vi "Roi_test.vi"() -> ()   [LabVIEW 2021]
panel:
  in  "Combo Box":string(combo)
  out "Image 2":T1(plugin-control)
  in  "stop":bool
  in  "input image":path
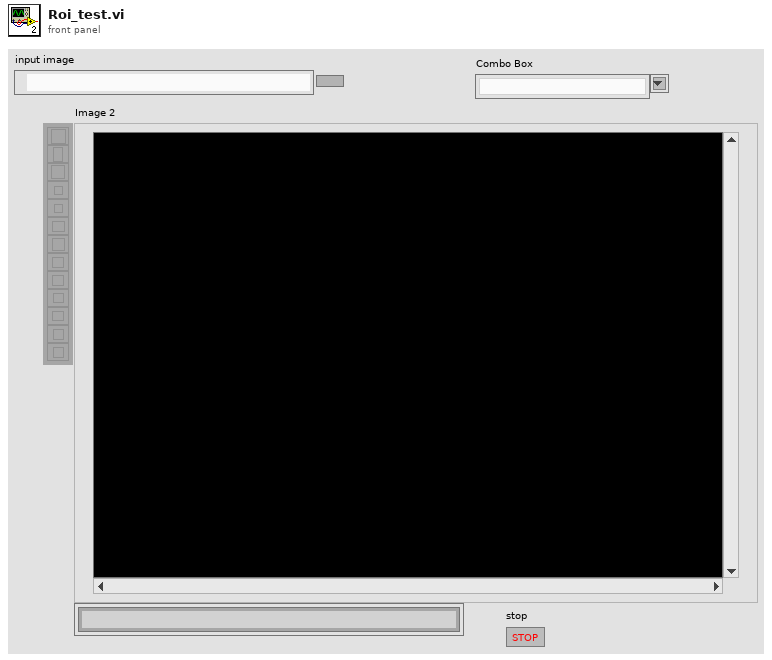
[diagram p1: front panel]
types:
  T1 = typedef "IMAQ Image.ctl" = refnum<image>
  T2 = typedef "Image Type" = u32
  T3 = cluster{"Desired Font (Application)":enum16{"User-specified Font", "Application Font", "System Font", "Dialog Font"}, "[User-specified Font]":cluster{"Font Name":string, "Size":i16, "Strikeout?":bool, "Italic?":bool, "Underline?":bool, "Outline?":bool, "Shadow?":bool, "Bold?":bool, "Rotation Angle":dbl}, "Horizontal Alignment":i16, "Vertical Alignment":i16}
  T4 = cluster{"Global Rectangle":i32[], "Contours":cluster{"Contour Type":u32, "ROI Type":u32, "Points":i32[]}[]}
  T5 = cluster{"Contour Type":u32, "ROI Type":u32, "Points":i32[]}[]
  T6 = cluster{"Contour Type":u32, "ROI Type":u32, "Points":i32[]}
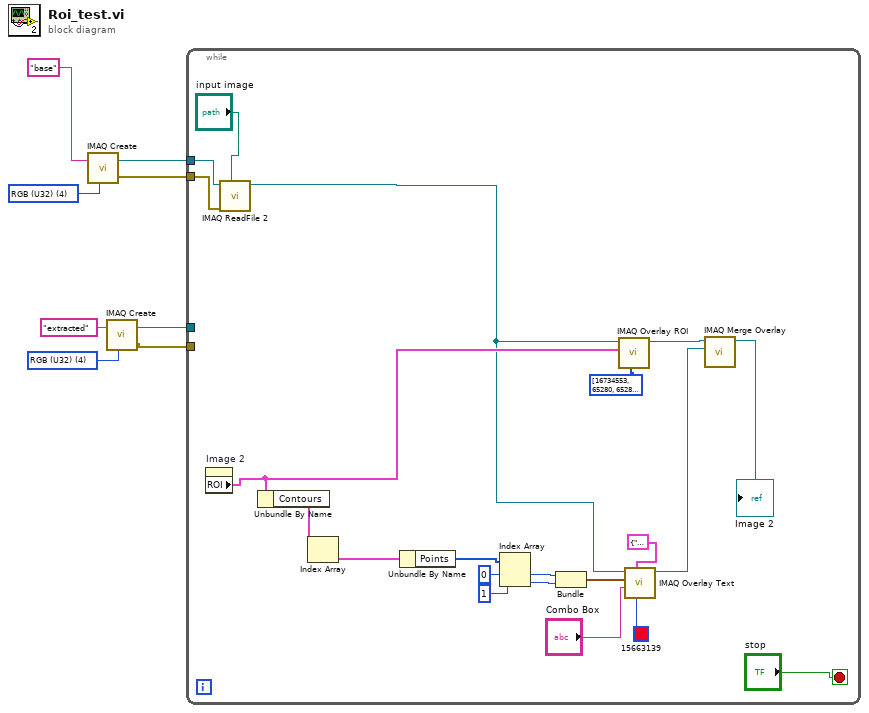
[diagram p0: block diagram]
diagram:
  w1 = T2 4 items=["Grayscale (U8)", "Grayscale (I16)", "Grayscale (SGL)", "Complex (CSG)", "RGB (U32)", "HSL (U32)", "RGB (U64)", "Grayscale (U16)"] ("Image Type")
  w2 = T2 4 items=["Grayscale (U8)", "Grayscale (I16)", "Grayscale (SGL)", "Complex (CSG)", "RGB (U32)", "HSL (U32)", "RGB (U64)", "Grayscale (U16)"] ("Image Type")
  n1 = call "IMAQ Create"("Image Name"="base", "Image Type"=w2) -> ("New Image"=w6:T1, "error out"=w7:errorcluster)  [unwired: 3 in]
  n2 = call "IMAQ Create"("Image Name"="extracted", "Image Type"=w1) -> ("New Image"=w5:T1, "error out"=w4:errorcluster)  [unwired: 3 in]
  n3 = while {
    tunnel: w7 -> [w29]
    tunnel: w6 -> [w28]
    tunnel: w5 -> [_]
    tunnel: w4 -> [_]
    stop <- "stop" stop-if-true
    n4 = property on="Image 2" class="ImageControl"() -> ("ROI"=w24:T4)  [unwired: 2 in, 2 out]
    n5 = call "IMAQ ReadFile 2"("File Path"="input image", "error in (no error)"=w29, "Image"=w28) -> ("Image Out"=w22:T1)  [unwired: 4 in, 4 out]
    n6 = Unbundle By Name(w24) -> ("Contours"=w19:T5)
    n7 = Index Array(array=w19) -> (element=w18:T6)  [unwired: 1 in]
    n8 = Unbundle By Name(w18) -> ("Points"=w17:i32[])
    n9 = Index Array(array=w17, index #1=0 ("index"), index #2=1 ("index")) -> (element #1=w13:i32, element #2=w14:i32)
    n10 = Bundle(w13, w14) -> (w12:cluster{i32, i32})  [unwired: 1 in]
    n11 = call "IMAQ Overlay ROI"("Colors (Green)"=u32[] [16734553, 65280, 65280, 16722479], "ROI Descriptor"=w24, "Image"=w22) -> ("Image Out"=w10:T1)  [unwired: 7 in, 1 out]
    n12 = call "IMAQ Overlay Text"("Text Color (black)"=u32 15663139, "Font, Size & Style"=T3 {"Desired Font (Application)"=enum."Application Font", "[User-specified Font]"={"Font Name"="", "Size"=40, "Strikeout?"=FALSE, "Italic?"=FALSE, "Underline?"=FALSE, "Outline?"=FALSE, "Shadow?"=FALSE, "Bold?"=FALSE, "Rotation Angle"=0.0}, "Horizontal Alignment"=0, "Vertical Alignment"=0}, "String"="Combo Box", "Origin"=w12, "Image"=w22) -> ("Image Out"=w9:T1)  [unwired: 5 in, 1 out]
    n13 = call "IMAQ Merge Overlay"("Image Dst"=w9, "Image Src"=w10) -> ("Image Dst Out"=→"Image 2":T1)  [unwired: 8 in, 1 out]
  }
